vi "Start Timer.vi"(0 "reference in":refnum<class "Timer.lvclass">, 5 "error in (no error)":errorcluster) -> (14 "reference out":refnum<class "Timer.lvclass">, 19 "error out":errorcluster)   [LabVIEW 2017, in "Timer.lvclass"]
uses:
  Timer.lvclass
  utils/Timer_Run.vi
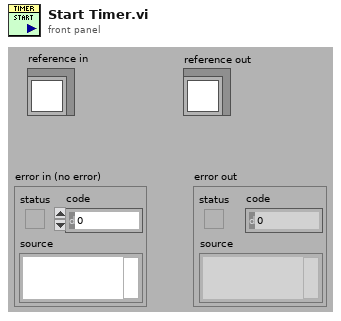
[diagram p1: front panel]
types:
  T1 = typedef "Timer.lvclass/ObjectAttributes.ctl" = cluster{"Timer is Timing":bool, "Timer Time (ms)":u32, "Timer VI Reference":refnum<vi>}
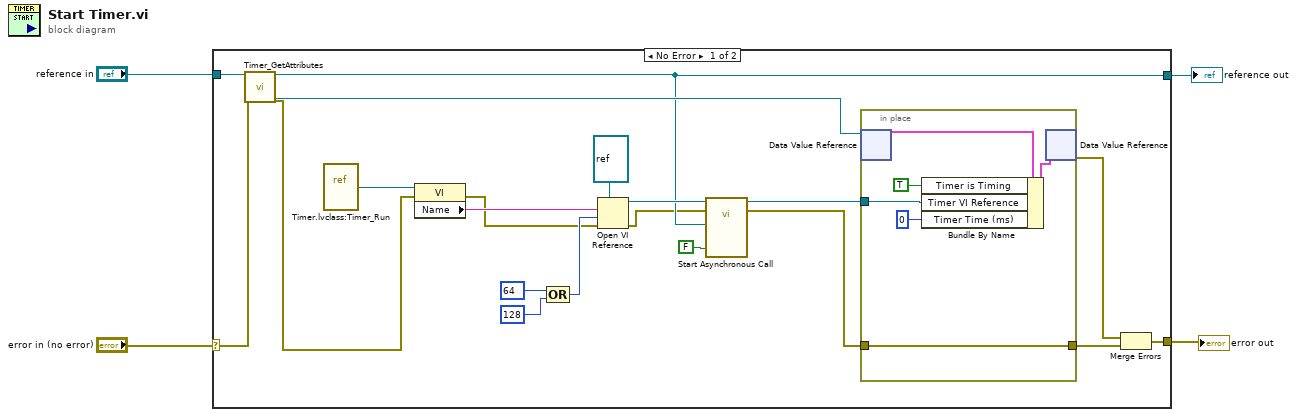
[diagram p0: block diagram]
diagram:
  n1 = case shown="No Error" "error in (no error)" {
    selector: "error in (no error)" -> [w23 w32]
    tunnel: [w22 w32] -> w3
    tunnel: [w16 w31] -> w1
    tunnel: "reference in" -> [w24 w31]
    frame No Error {
      n2 = call "Timer_GetAttributes.vi"("reference in"=w24, "error in (no error)"=w23) -> ("reference out"=w16:refnum<class "Timer.lvclass">, "DataRef"=w21:refnum<data-value>, "error out"=w5:errorcluster)  [unwired: 14 in, 1 out]
      n3 = vi-ref "Timer.lvclass:Timer_Run.vi"() -> (w14:refnum<vi>)
      n4 = property class="VI"(reference=w14, error in=w5) -> (error out=w8:errorcluster, "Name"=w15:string)  [unwired: 1 out]
      n5 = Compound Arithmetic op=OR(64 ("options"), 128 ("options")) -> (w11:i32)
      n6 = Open VI Reference(type specifier VI Refnum (for type only)=refnum<vi> refnum, vi path=w15, options=w11, error in (no error)=w8) -> (vi reference=w17:refnum<vi>, error out=w7:errorcluster)  [unwired: 2 in]
      n7 = call-by-ref "Start Asynchronous Call"(reference=w17, error in=w7, "Stop Timer"=FALSE, "reference in"=w16) -> (reference out=w12:refnum<vi>, error out=w6:errorcluster)  [unwired: 9 in, 1 out]
      n8 = in-place {
        in-place-border: w6 -> [w28]
        in-place-border: [w28] -> w19
        in-place-border: w12 -> [w26]
        n9 = in-place-dvr #1(w21) -> (w29:T1)  [unwired: 1 out]
        n10 = Bundle By Name(cluster=w29, "Timer is Timing"=TRUE ("Timer Status (On/Off)"), "Timer VI Reference"=w26, "Timer Time (ms)"=u32 0) -> (w30:T1)
        n11 = in-place-dvr #1(w30) -> (w20:errorcluster)  [unwired: 1 out]
      }
      n12 = Merge Errors(w20, w19) -> (w22:errorcluster)
    }
    frame Error {
    }
  }
  "error out" <- w3
  "reference out" <- w1
